vi "相机频率测试.vi"() -> ()   [LabVIEW 2017]
uses:
  <vilib>/vision/driver/NI_Vision_Acquisition_Software.lvlib
  <vilib>/userdefined/High Color/IMAQdx.ctl
panel:
  out "acquired FPS":dbl
  in  "Camera Name":T1
  in  "stop":bool
  out "Frame Rate":dbl(knob) scale=0.0..210.0 scale format="%.1f"
  out "Image":T2(plugin-control)
  out "Buffer Number":u32
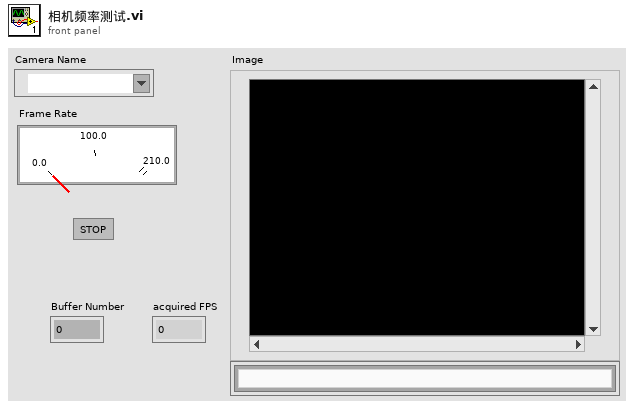
[diagram p1: front panel]
types:
  T1 = typedef "IMAQdx.ctl" = refnum<k21>
  T2 = typedef "IMAQ Image.ctl" = refnum<image>
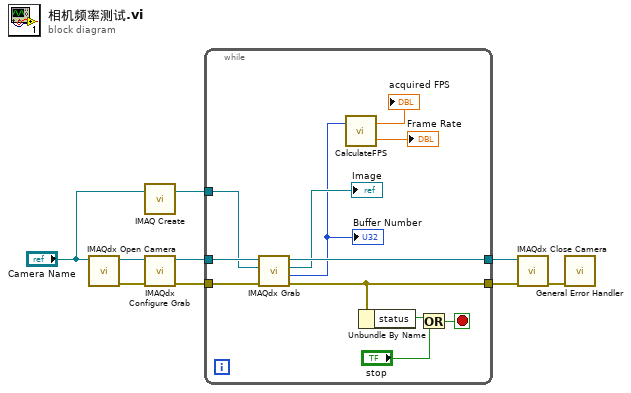
[diagram p0: block diagram]
diagram:
  n1 = call <vilib>:"IMAQdx Open Camera.vi"("Session In"="Camera Name") -> ("error out"=w3:errorcluster, "Session Out"=w2:T1)  [unwired: 2 in, 7 out]
  n2 = call "IMAQ Create"("Image Name"="Camera Name") -> ("New Image"=w9:T2)  [unwired: 3 in, 2 out]
  n3 = call <vilib>:"IMAQdx Configure Grab.vi"("error in"=w3, "Session In"=w2) -> ("error out"=w7:errorcluster, "Session Out"=w8:T1)  [unwired: 8 out]
  n4 = while {
    tunnel: [w15] -> w6
    tunnel: w7 -> [w17]
    tunnel: w8 -> [w18]
    tunnel: [w14] -> w5
    tunnel: w9 -> [w16]
    stop <- w21 stop-if-true
    n5 = call <vilib>:"IMAQdx Grab.vi"("error in"=w17, "Image In"=w16, "Session In"=w18) -> ("error out"=w14:errorcluster, "Buffer Number Out"=w11:u32, "Image Out"=→"Image":T2, "Session Out"=w15:T1)  [unwired: 1 in, 4 out]
    "Buffer Number" <- w11
    n6 = call "CalculateFPS.vi"("buffer number"=w11) -> ("processed FPS"=→"Frame Rate":dbl, "acquired FPS"=→"acquired FPS":dbl)  [unwired: 1 out]
    n7 = Unbundle By Name(w14) -> ("status"=w20:bool)
    n8 = Or(x=w20, y="stop") -> (x .or. y?=w21:bool)
  }
  n9 = call <vilib>:"IMAQdx Close Camera.vi"("error in"=w5, "Session In"=w6) -> ("error out"=w4:errorcluster)  [unwired: 9 out]
  n10 = call <vilib>:"General Error Handler.vi"("error in (no error)"=w4) -> ()  [unwired: 2 in, 13 out]
